vi "DSF.Engine.Framework.Initialize.vi"(8 "error in (no error)":errorcluster, 10 "Framework Configuration":refnum<class "DSF.Shared.Configuration.Framework.lvclass">, 11 "Framework type":refnum<class "DSF.Engine.Framework.lvclass">) -> (0 "error out":errorcluster, 3 "Framework out":refnum<class "DSF.Engine.Framework.lvclass">)   [LabVIEW 2017, in "DSF.Engine.lvlib" / "DSF.Engine.Framework.lvclass"]
uses:
  DSF.Engine.Framework.lvclass
  Shared/Classes/Framework/DSF.Shared.Configuration.Framework.lvclass
  Transceiver/DSF.Engine.Transceiver Loader.lvclass
  DSF.Engine.Framework.lvclass/DSF.Engine.Framework.ctl
  Shared/Classes/Framework/DSF.Shared.Configuration.Framework.lvclass/DSF.Shared.Configuration.Framework.ctl
  Status/DSF.Engine.Status.Framework.lvclass
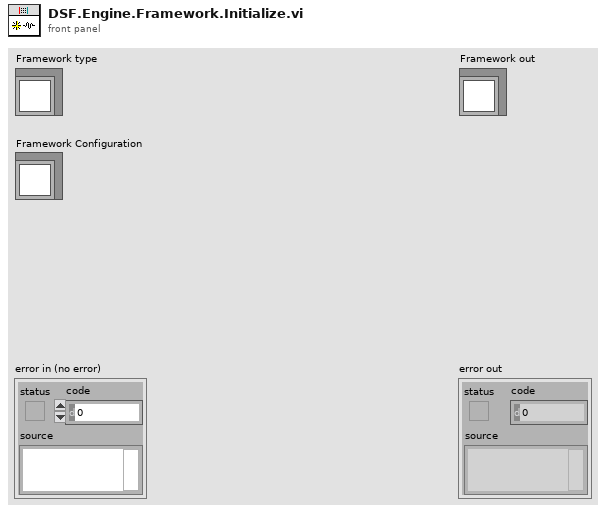
[diagram p1: front panel]
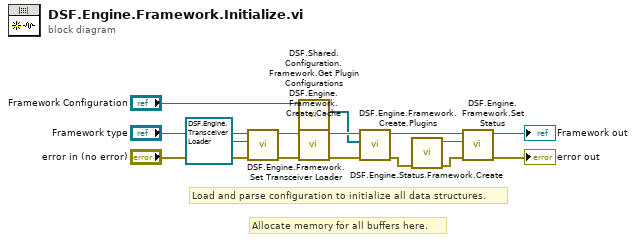
[diagram p0: block diagram]
diagram:
  # "Allocate memory for all buffers here."
  # "Load and parse configuration to initialize all data structures."
  n1 = call "DSF.Engine.Framework.Set Transceiver Loader.vi"("Transceiver Loader"=refnum<class "DSF.Engine.Transceiver Loader.lvclass"> refnum, "Framework in"="Framework type") -> ("Framework out"=w2:refnum<class "DSF.Engine.Framework.lvclass">)  [unwired: 9 in]
  n2 = call "DSF.Shared.Configuration.Framework.Get Plugin Configurations.vi"("Framework Configuration in"="Framework Configuration") -> ("Plugin Configurations"=w9:refnum<class "DSF.Shared.Configuration.Plugin.lvclass">[])  [unwired: 9 in, 1 out]
  n3 = call "DSF.Engine.Framework.Create.Cache.vi"("error in (no error)"="error in (no error)", "Framework in"=w2) -> ("error out"=w10:errorcluster, "Framework out"=w11:refnum<class "DSF.Engine.Framework.lvclass">)  [unwired: 8 in]
  n4 = call "DSF.Engine.Framework.Create.Plugins.vi"("error in (no error)"=w10, "Plugin Configurations"=w9, "Framework in"=w11) -> ("error out"=w8:errorcluster, "Framework out"=w5:refnum<class "DSF.Engine.Framework.lvclass">)  [unwired: 6 in, 1 out]
  n5 = call "DSF.Engine.Status.Framework.Create.vi"("error in (no error)"=w8) -> ("error out"=→"error out":errorcluster, "Framework Status"=w6:refnum<class "DSF.Engine.Status.Framework.lvclass">)  [unwired: 9 in]
  n6 = call "DSF.Engine.Framework.Set Status.vi"("Status"=w6, "Framework in"=w5) -> ("Framework out"=→"Framework out":refnum<class "DSF.Engine.Framework.lvclass">)  [unwired: 9 in]
